vi "Batch Channel Settings Dialog.vi"(8 "error in (no error)":errorcluster, 9 "Data Entry Limits:Maximum":dbl) -> (0 "error out":errorcluster, 1 "scaling information":variant, 2 "# of Chans":u8, 3 "bridge information":variant, 4 "Maximum Value":T3, 5 "Sensor Type":T1, 6 "Minimum Value":T2)   [LabVIEW 2010, in "PXIe-433x Custom Device.lvlib"]
uses:
  PXIe-433x Custom Device.lvlib
  Max Value.ctl
  Min Value.ctl
  Sensor Type.ctl
  Force Props.vi
  Pressure Props.vi
  Torque Props.vi
panel:
  in  "Type of Channels to Add":T1
  in  "OK":bool
  in  "Number of Channels To Add?":u8=8 max=0 step=1
  # "Default Channel Settings"
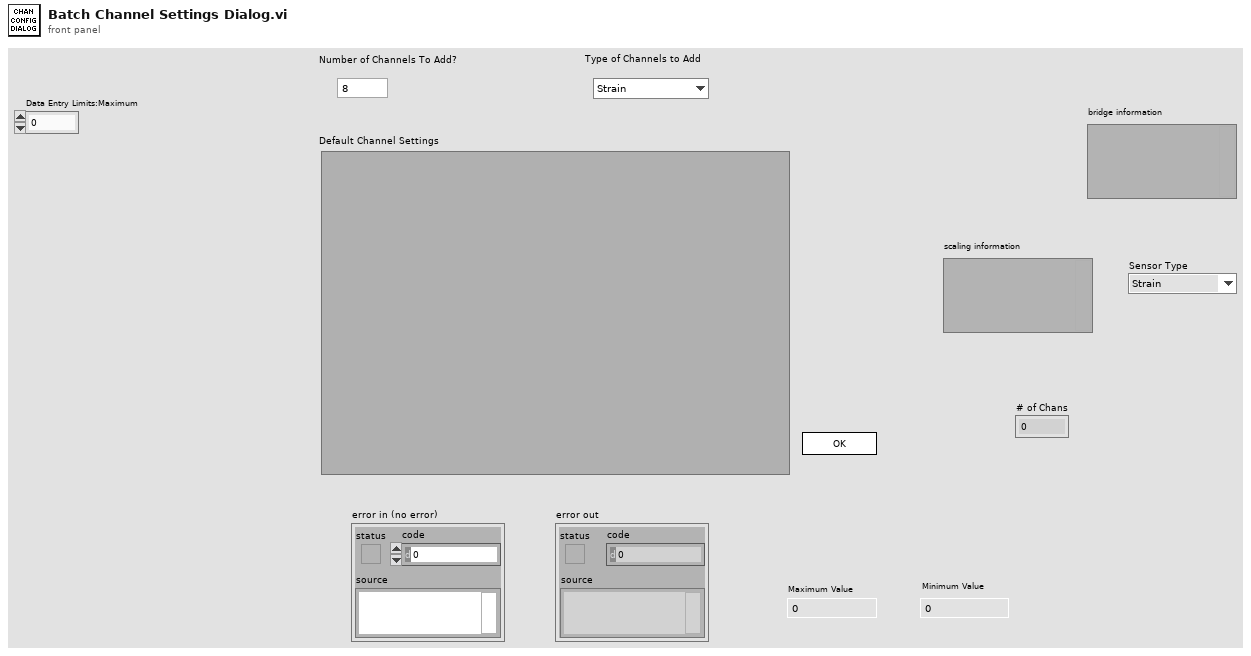
[diagram p1: front panel]
types:
  T1 = typedef "PXIe-433x Custom Device.lvlib/Sensor Type.ctl" = enum16{"Strain", "Force", "Pressure", "Torque"}
  T2 = typedef "PXIe-433x Custom Device.lvlib/Min Value.ctl" = dbl
  T3 = typedef "PXIe-433x Custom Device.lvlib/Max Value.ctl" = dbl
  T4 = typedef "PXIe-433x Custom Device.lvlib/Board Info for checking settings.ctl" = cluster{"Present?":bool, "Created by CD code?":bool, "Resource Name":string}
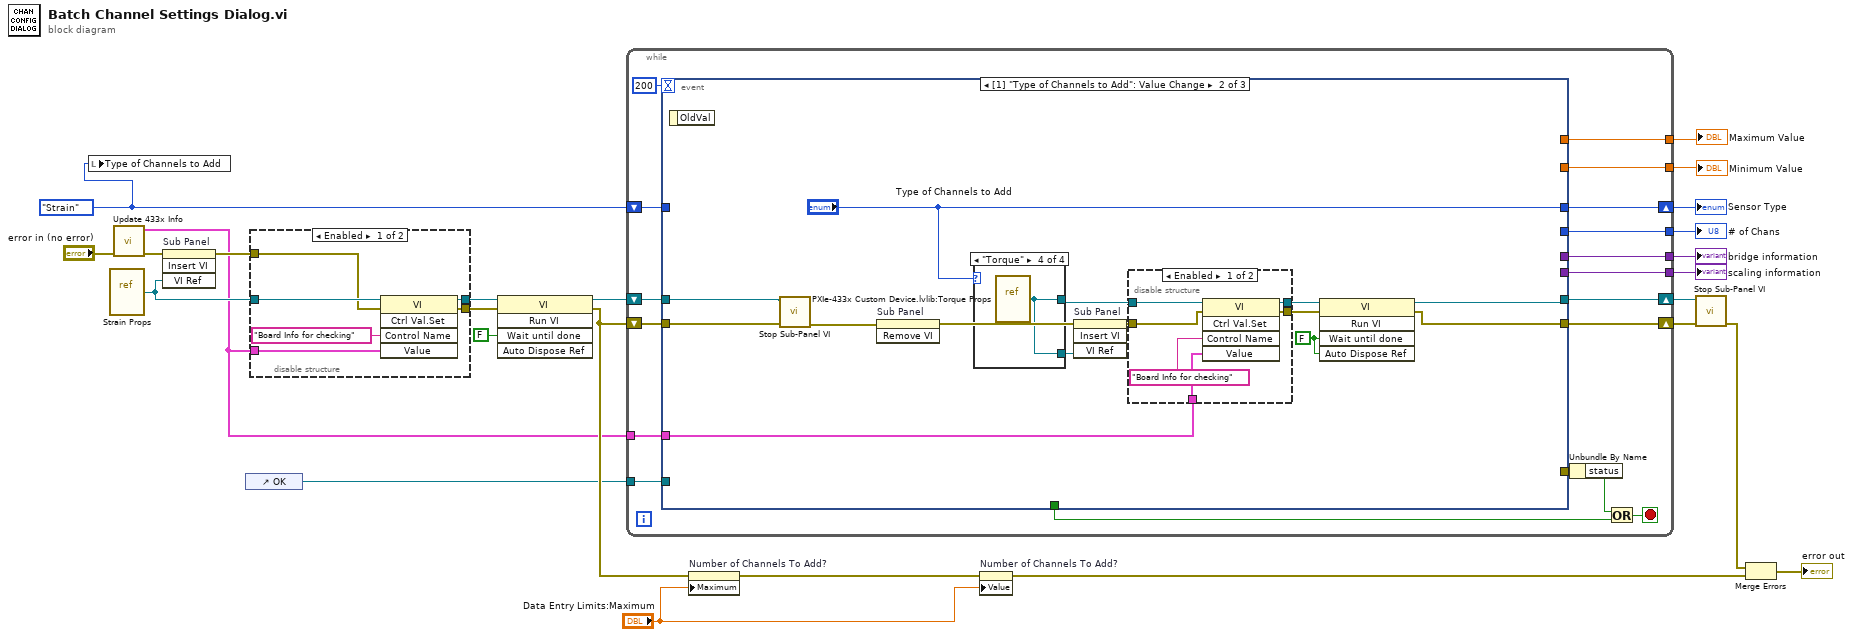
[diagram p0: block diagram]
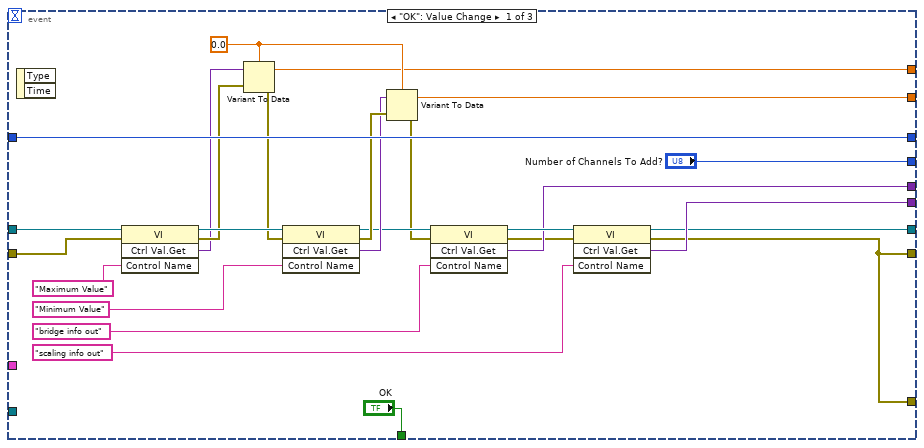
[diagram p3: hidden frame]
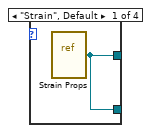
[diagram p5: hidden frame]
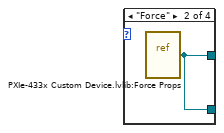
[diagram p6: hidden frame]
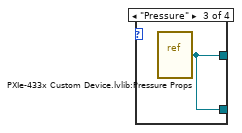
[diagram p7: hidden frame]
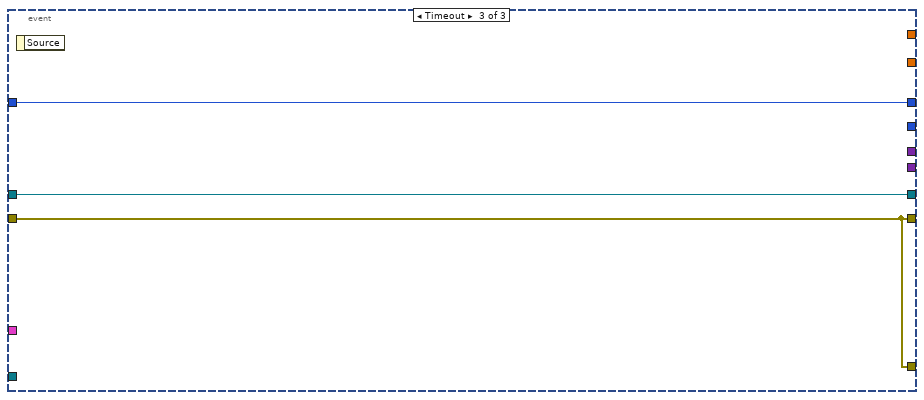
[diagram p8: hidden frame]
diagram:
  w15 = Sensor_Type."Strain" ("Type of Channels to Add")
  n1 = local write "Type of Channels to Add"(w15) -> ()
  n2 = vi-ref "Strain Props.vi"() -> (w22:refnum<vi>)
  n3 = call "Update 433x Info.vi"("error in (no error)"="error in (no error)") -> ("error IO"=w2:errorcluster, "Board Info for checking"=w1:T4)  [unwired: 9 in]
  n4 = invoke on="Sub Panel" class="SubPnl" method="Insert VI"(error in=w2, "VI Ref"=w22) -> (error out=w11:errorcluster)  [unwired: 2 in, 3 out]
  n5 = control-ref of="OK"() -> (w9:refnum<vi>)
  n6 = disable-structure shown="Enabled" {
    disable-tunnel: w22 -> [w31 w33]
    disable-tunnel: [w30 w33] -> w12
    disable-tunnel: w11 -> [w29 w32]
    disable-tunnel: [w28 w32] -> w10
    disable-tunnel: w1 -> [w26 _]
    frame Enabled {
      n7 = invoke class="VI" method="Ctrl Val.Set"(reference=w31, error in=w29, "Control Name"="Board Info for checking", "Value"=w26) -> (reference out=w30:refnum<vi>, error out=w28:errorcluster)  [unwired: 1 in, 3 out]
    }
    frame Disabled {
    }
  }
  n8 = invoke class="VI" method="Run VI"(reference=w12, error in=w10, "Wait until done"=FALSE ("Wait Until Done")) -> (reference out=w14:refnum<vi>, error out=w13:errorcluster)  [unwired: 2 in, 3 out]
  n9 = while {
    tunnel: [w51] -> w25
    shift-right: [w45] -> w19
    shift-left: w13 -> [w49]
    shift-right: [w43] -> w16
    shift-left: w15 -> [w42]
    shift-right: [w48] -> w17
    shift-left: w14 -> [w50]
    tunnel: w9 -> [w41]
    tunnel: [w40] -> w7
    tunnel: [w39] -> w6
    tunnel: [w38] -> w5
    tunnel: [w37] -> w4
    tunnel: w1 -> [w34]
    stop <- w46 stop-if-true
    n10 = event shown="[1] \"Type of Channels to Add\": Value Change" {
      selector: _ -> [_ _ _]
      dyn-events: _ -> [_ _ _]
      timeout: 200 -> [_ _ _]
      tunnel: ["Number of Channels To Add?" _ _] -> w51
      tunnel: w50 -> [w74 w81 w105]
      tunnel: w49 -> [w73 w79 w104]
      tunnel: [w52 w83 w104] -> w45
      tunnel: [w53 w85 w105] -> w48
      tunnel: ["OK" _ _] -> w47
      tunnel: [w75 "Type of Channels to Add" w106] -> w43
      tunnel: w42 -> [w75 _ w106]
      tunnel: w41 -> [_ _ _]
      tunnel: [w63 _ _] -> w40
      tunnel: [w62 _ _] -> w39
      tunnel: [w57 _ _] -> w38
      tunnel: [w54 _ _] -> w37
      tunnel: [w52 _ w104] -> w36
      tunnel: w34 -> [_ w78 _]
      event "OK": Value Change {
        w66 = 0.0
        n11 = event-data() -> ()  [unwired: 1 in, 2 out]
        n12 = invoke class="VI" method="Ctrl Val.Get"(reference=w74, error in=w73, "Control Name"="Maximum Value") -> (reference out=w71:refnum<vi>, error out=w69:errorcluster, "Get Control Value Variant"=w68:variant)  [unwired: 1 in, 1 out]
        n13 = Variant To Data(error in=w69, Variant=w68, type=w66) -> (error out=w67:errorcluster, data=w63:dbl)
        n14 = invoke class="VI" method="Ctrl Val.Get"(reference=w71, error in=w67, "Control Name"="Minimum Value") -> (reference out=w61:refnum<vi>, error out=w65:errorcluster, "Get Control Value Variant"=w64:variant)  [unwired: 1 in, 1 out]
        n15 = Variant To Data(error in=w65, Variant=w64, type=w66) -> (error out=w60:errorcluster, data=w62:dbl)
        n16 = invoke class="VI" method="Ctrl Val.Get"(reference=w61, error in=w60, "Control Name"="bridge info out") -> (reference out=w58:refnum<vi>, error out=w56:errorcluster, "Get Control Value Variant"=w57:variant)  [unwired: 1 in, 1 out]
        n17 = invoke class="VI" method="Ctrl Val.Get"(reference=w58, error in=w56, "Control Name"="scaling info out") -> (reference out=w53:refnum<vi>, error out=w52:errorcluster, "Get Control Value Variant"=w54:variant)  [unwired: 1 in, 1 out]
      }
      event Value Change {
        w89 = FALSE ("Wait Until Done")
        n18 = event-data() -> ()  [unwired: 1 in, 1 out]
        n19 = call "Stop Sub-Panel VI.vi"("error in (no error) 2"=w79, "reference"=w81) -> ("error IO"=w80:errorcluster)  [unwired: 9 in]
        n20 = invoke on="Sub Panel" class="SubPnl" method="Remove VI"(error in=w80) -> (error out=w82:errorcluster)  [unwired: 2 in, 2 out]
        n21 = case shown="\"Torque\"" "Type of Channels to Add" {
          tunnel: [w100 w101 w102 w103] -> w88
          tunnel: [w100 w101 w102 w103] -> w91
          frame "Strain", Default {
            n22 = vi-ref "Strain Props.vi"() -> (w100:refnum<vi>)
          }
          frame "Force" {
            n23 = vi-ref "PXIe-433x Custom Device.lvlib:Force Props.vi"() -> (w101:refnum<vi>)
          }
          frame "Pressure" {
            n24 = vi-ref "PXIe-433x Custom Device.lvlib:Pressure Props.vi"() -> (w102:refnum<vi>)
          }
          frame "Torque" {
            n25 = vi-ref "PXIe-433x Custom Device.lvlib:Torque Props.vi"() -> (w103:refnum<vi>)
          }
        }
        n26 = invoke on="Sub Panel" class="SubPnl" method="Insert VI"(error in=w82, "VI Ref"=w91) -> (error out=w84:errorcluster)  [unwired: 2 in, 3 out]
        n27 = disable-structure shown="Enabled" {
          disable-tunnel: w84 -> [w96 w98]
          disable-tunnel: w88 -> [w95 w99]
          disable-tunnel: [w94 w99] -> w87
          disable-tunnel: [w93 w98] -> w86
          disable-tunnel: w78 -> [w92 _]
          frame Enabled {
            n28 = invoke class="VI" method="Ctrl Val.Set"(reference=w95, error in=w96, "Control Name"="Board Info for checking", "Value"=w92) -> (reference out=w94:refnum<vi>, error out=w93:errorcluster)  [unwired: 1 in, 3 out]
          }
          frame Disabled {
          }
        }
        n29 = invoke class="VI" method="Run VI"(reference=w87, error in=w86, "Wait until done"=w89, "Auto Dispose Ref"=w89) -> (reference out=w85:refnum<vi>, error out=w83:errorcluster)  [unwired: 1 in, 3 out]
      }
      event Timeout {
        n30 = event-data() -> ()  [unwired: 1 in, 1 out]
      }
    }
    n31 = Unbundle By Name(w36) -> ("status"=w44:bool)
    n32 = Or(x=w44, y=w47) -> (x .or. y?=w46:bool)
  }
  "# of Chans" <- w25
  "Maximum Value" <- w7
  "Minimum Value" <- w6
  "bridge information" <- w5
  "scaling information" <- w4
  "Sensor Type" <- w16
  n33 = property on="Number of Channels To Add?" class="DigNum (strict)"(error in=w13, "Maximum"="Data Entry Limits:Maximum") -> (error out=w23:errorcluster)  [unwired: 1 in, 1 out]
  n34 = property on="Number of Channels To Add?" class="DigNum (strict)"(error in=w23, "Value"="Data Entry Limits:Maximum") -> (error out=w20:errorcluster)  [unwired: 1 in, 1 out]
  n35 = call "Stop Sub-Panel VI.vi"("error in (no error) 2"=w19, "reference"=w17) -> ("error IO"=w18:errorcluster)  [unwired: 9 in]
  n36 = Merge Errors(w18, w20) -> (→"error out":errorcluster)
